vi "thermocouple_analog_input_multichannel_consumer.vi"(4 "Sampling Window [s]":dbl, 6 "Sampling Frequency [Hz]":dbl=2500.0, 7 "Number of Channels":i32, 8 "error in (no error)":errorcluster, 9 "Offset":dbl[](array[numeric]), 10 "Scale":dbl[](array[numeric]), 11 "queue out":refnum<queue>) -> (0 "error out":errorcluster, 1 "CJTemp[K]":dbl[](array[numeric]), 2 "TC [V]":dbl[](array[numeric]), 3 "TC [degC]":dbl[](array[numeric]))   [LabVIEW 2025, in "LabJackEKG.lvlib"]
uses:
  LabJackEKG.lvlib
  <vilib>/Analysis/baseanly.llb/Mean (DBL).vi
  <vilib>/Analysis/NI_AALBase.lvlib
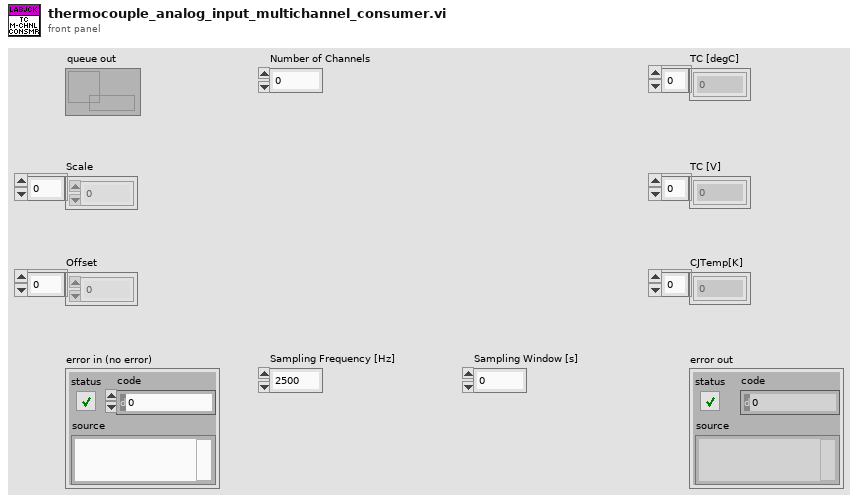
[diagram p1: front panel]
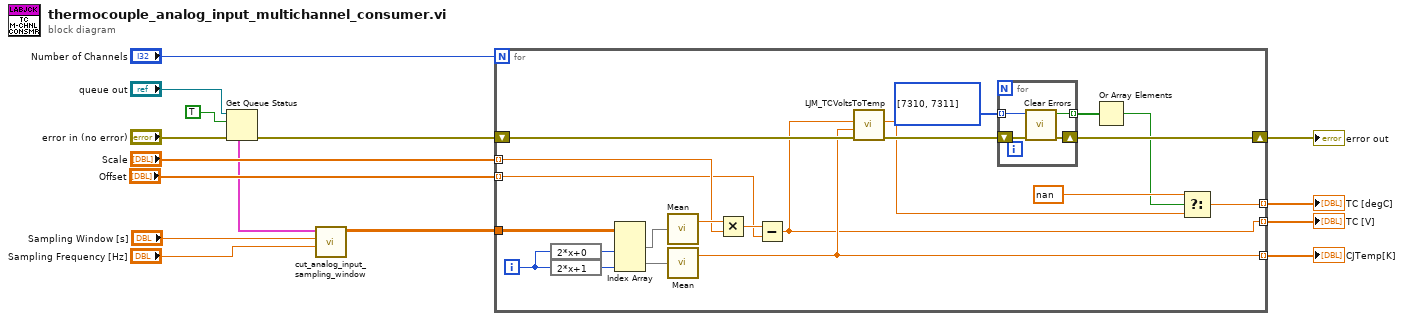
[diagram p0: block diagram]
diagram:
  n1 = Get Queue Status(queue="queue out", return elements? (F)=TRUE, error in (no error)="error in (no error)") -> (error out=w11:errorcluster, elements=w4:cluster{"Volt":dbl[]}[])  [unwired: 6 out]
  n2 = call "cut_analog_input_sampling_window.vi"("Sampling Frequency [Hz]"="Sampling Frequency [Hz]", "Sampling Window [s]"="Sampling Window [s]", "elements"=w4) -> ("Volt"=w3:dbl[][])  [unwired: 7 in, 1 out]
  n3 = for {
    N: "Number of Channels" -> [_]
    tunnel: w3 -> [w36]
    tunnel: [w25] -> w9 mode=indexing
    tunnel: [w21] -> w8 mode=indexing
    shift-right: [w18] -> w10
    shift-left: w11 -> [w27]
    tunnel: [w23] -> w7 mode=indexing
    tunnel: "Scale" -> [w20] mode=indexing
    tunnel: "Offset" -> [w19] mode=indexing
    i -> [w35]
    n4 = expression code="2*x+0"(w35) -> (w34:i32)
    n5 = expression code="2*x+1"(w35) -> (w33:i32)
    n6 = Index Array(array=w36, index (col) #1=w34, index (col) #2=w33) -> (element #1=w31:dbl[], element #2=w32:dbl[])  [unwired: 2 in]
    n7 = call-poly <vilib>:"Mean.vi"("X"=w31) -> ("mean"=w24:dbl)  [unwired: 1 out]
    n8 = call-poly <vilib>:"Mean.vi"("X"=w32) -> ("mean"=w23:dbl)  [unwired: 1 out]
    n9 = Multiply(x=w24, y=w20) -> (x*y=w22:dbl)
    n10 = Subtract(x=w22, y=w19) -> (x-y=w21:dbl)
    n11 = call <vilib>:"LJM_TCVoltsToTemp.vi"("error in"=w27, "CJTempK"=w23, "TCVolts"=w21) -> ("error out"=w26:errorcluster, "TCTempC"=w16:dbl)  [unwired: 5 in, 2 out]
    n12 = for {
      tunnel: [w40] -> w30 mode=indexing
      tunnel: i32[] [7310, 7311] ("specific error code to clear (0: all)") -> [w39] mode=indexing
      shift-right: [w37] -> w18
      shift-left: w26 -> [w38]
      n13 = call <vilib>:"Clear Errors.vi"("error in (no error)"=w38, "specific error code to clear (0: all)"=w39) -> ("error out"=w37:errorcluster, "specific error cleared?"=w40:bool)  [unwired: 4 in]
    }
    n14 = Or Array Elements(Boolean array=w30) -> (logical OR=w17:bool)
    n15 = Select(t=nan, s=w17, f=w16) -> (s? t:f=w25:dbl)
  }
  "error out" <- w10
  "TC [degC]" <- w9
  "TC [V]" <- w8
  "CJTemp[K]" <- w7
